vi "pmu_Check Reporting Rate Error.vi"(8 "error in (no error)":errorcluster, 10 "reporting rate":i16=60, 11 "nominal frequency":enum16{"50 Hz", "60 Hz"}(ring)=enum."60 Hz") -> (0 "error out":errorcluster)   [LabVIEW 2011, in "NI_EP_PMU.lvlib"]
uses:
  <vilib>/addons/Electrical Power/PMU/NI_EP_PMU.lvlib
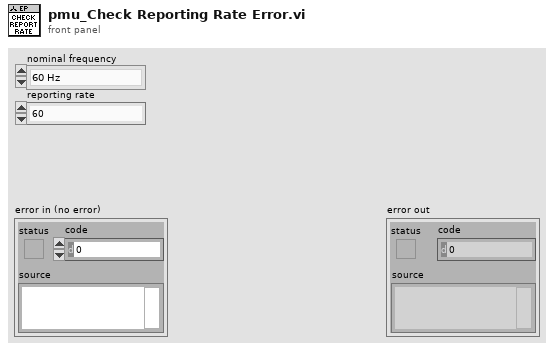
[diagram p1: front panel]
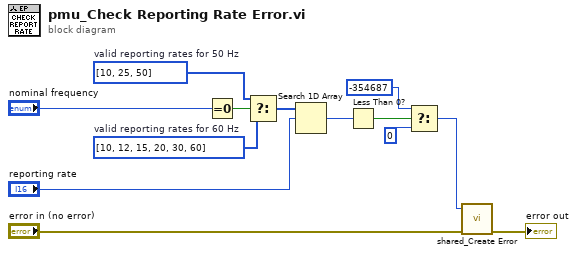
[diagram p0: block diagram]
diagram:
  w11 = i16[] [10, 25, 50]  # valid reporting rates for 50 Hz
  w10 = i16[] [10, 12, 15, 20, 30, 60]  # valid reporting rates for 60 Hz
  n1 = Equal To 0?(x="nominal frequency") -> (x = 0?=w13:bool)
  n2 = Select(t=w11, s=w13, f=w10) -> (s? t:f=w9:i16[])
  n3 = Search 1D Array(1D array=w9, element="reporting rate") -> (index of element=w7:i32)  [unwired: 1 in]
  n4 = Less Than 0?(x=w7) -> (x < 0?=w6:bool)
  n5 = Select(t=-354687 ("error code (0)"), s=w6, f=0 ("error code (0)")) -> (s? t:f=w1:i32)
  n6 = call <vilib>:"shared_Create Error.vi"("error in (no error)"="error in (no error)", "error code (0)"=w1) -> ("error out"=→"error out":errorcluster)  [unwired: 9 in]
